vi "CSTK_Icon_Creator_CreateLogo_InputImage.vi"(8 "错误输入（无错误）":errorcluster, 10 "LOGO图像路径":path, 11 "LOGO输入":refnum<vi>) -> (0 "错误输出":errorcluster, 3 "LOGO输出":refnum<vi>)   [LabVIEW 2015, in "CSTK_Icon Creator.lvlib"]
uses:
  CSTK_Icon Creator.lvlib
  <vilib>/picture/picture.llb/Draw True-Color Pixmap.vi
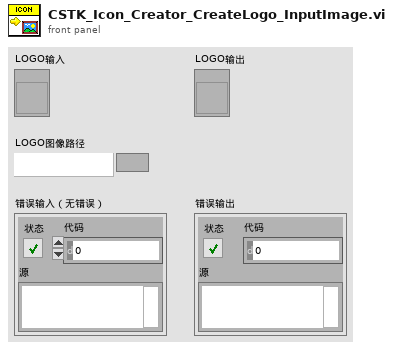
[diagram p1: front panel]
types:
  T1 = typedef "imagedata.ctl" = cluster{"image type":i32, "image depth":i32, "image":u8[], "mask":u8[], "colors":u32[], "Rectangle":cluster{"left":i16, "top":i16, "right":i16, "bottom":i16}}
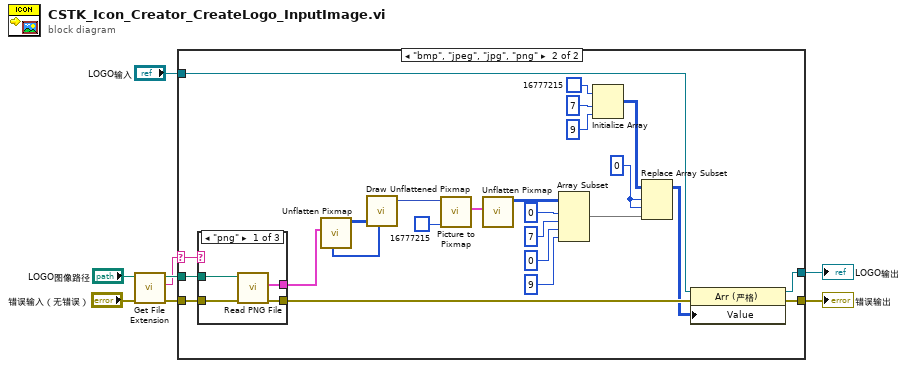
[diagram p0: block diagram]
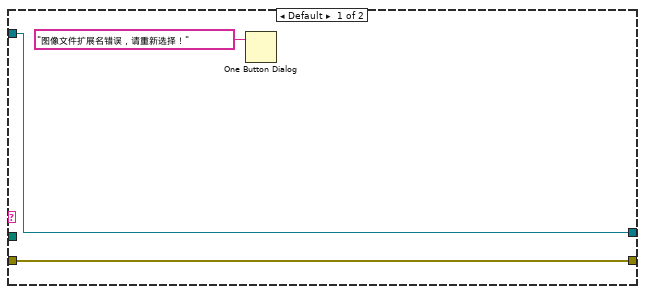
[diagram p2: hidden frame]
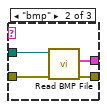
[diagram p3: hidden frame]
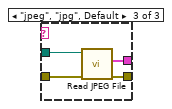
[diagram p4: hidden frame]
diagram:
  n1 = call <vilib>:"Get File Extension.vi"("error in (no error)"="错误输入（无错误）", "file"="LOGO图像路径") -> ("error out"=w7:errorcluster, "lowercase file extension"=w4:string, "dup file"=w5:path)  [unwired: 5 in, 2 out]
  n2 = case shown="\"bmp\", \"jpeg\", \"jpg\", \"png\"" w4 {
    selector: w4 -> [_ w36]
    tunnel: w5 -> [_ w35]
    tunnel: [w10 w18] -> w6
    tunnel: w7 -> [w10 w34]
    tunnel: "LOGO输入" -> [w9 w22]
    tunnel: [w9 w19] -> w1
    frame Default {
      n3 = One Button Dialog(message="图像文件扩展名错误，请重新选择！" ("消息")) -> ()  [unwired: 1 in, 1 out]
    }
    frame "bmp", "jpeg", "jpg", "png" {
      w24 = 0 ("索引 (行)")
      n4 = case shown="\"png\"" w36 {
        tunnel: w35 -> [w40 w44 w48]
        tunnel: w34 -> [w39 w43 w47]
        tunnel: [w38 w41 w45] -> w33
        tunnel: [w37 w42 w46] -> w21
        frame "png" {
          n5 = call <vilib>:"Read PNG File.vi"("error in (no error)"=w39, "path to PNG file"=w40) -> ("error out"=w37:errorcluster, "image data"=w38:T1)  [unwired: 7 in, 1 out]
        }
        frame "bmp" {
          n6 = call <vilib>:"Read BMP File.vi"("error in (no error)"=w43, "path to BMP file"=w44) -> ("error out"=w42:errorcluster, "image data"=w41:T1)  [unwired: 7 in, 1 out]
        }
        frame "jpeg", "jpg", Default {
          n7 = call <vilib>:"Read JPEG File.vi"("error in (no error)"=w47, "path to JPEG file"=w48) -> ("error out"=w46:errorcluster, "image data"=w45:T1)  [unwired: 7 in, 1 out]
        }
      }
      n8 = call <vilib>:"Unflatten Pixmap.vi"("image data"=w33) -> ("24-bit pixmap"=w17:u32[][], "mask"=w16:u8[])  [unwired: 4 in, 5 out]
      n9 = call-poly <vilib>:"Draw Unflattened Pixmap.vi"("data (RGB format)"=w17, "mask"=w16) -> ("new picture"=w15:picture)  [unwired: 7 in]
      n10 = call <vilib>:"Picture to Pixmap.vi"("Background Color"=u32 16777215, "picture"=w15) -> ("image data"=w13:T1)  [unwired: 8 in, 1 out]
      n11 = call <vilib>:"Unflatten Pixmap.vi"("image data"=w13) -> ("24-bit pixmap"=w12:u32[][])  [unwired: 4 in, 6 out]
      n12 = Array Subset(array=w12, index (row)=0 ("索引"), length (row)=7 ("长度"), index (col)=0 ("索引"), length (col)=9 ("长度")) -> (w23:u32[][])
      n13 = Initialize Array(u32 16777215, 7 ("维数大小"), 9 ("维数大小")) -> (w25:u32[][])
      n14 = Replace Array Subset(array=w25, new element=w23, index (row)=w24, index (col)=w24) -> (w20:u32[][])
      n15 = property class="Arr (严格)"(reference=w22, error in=w21, "Value"=w20) -> (reference out=w19:refnum<vi>, error out=w18:errorcluster)
    }
  }
  "错误输出" <- w6
  "LOGO输出" <- w1
